vi "testingImagesROI.vi"(8 "error in (no error)":errorcluster) -> (0 "error out":errorcluster)   [LabVIEW 2017]
doc: "Use this template to build a VI to use as a subVI."
uses:
  AEROTECstageAPI/SingleStageData.ctl
  AEROTECstageAPI/StageEnum.ctl
  AEROTECstageAPI/MoveDistanceInAxis.ctl
  Utility/Axis Direction Definition.ctl
  <vilib>/event_ctls.llb/lveventtype.ctl
  <vilib>/vision/NI_Vision_Development_Module.lvlib
panel:
  out "Number of Points":i32
  in  "Point Spacing (microns)":dbl(slide)=0.2 min=0.2 max=1000.0 scale=0.0..10.0
  in  "Clear Points":bool
  in  "File Path":path=path "C:/Users/OmerLab/Documents/GitHub/RamanSpecUsingStageXY/imagesForTesting/Snap-15.jpg"
  in  "Calibration Axis Info":T1={"Origin Pixel"={"X"=1232.0, "Y"=1028.0}, "Angle Relative to Horizontal (deg)"=0.0, "Axis Reference"=0} {"Axis Reference" items=["Direct", "Indirect"]; "Angle Relative to Horizontal (deg)" format="%.2f"; "Origin Pixel"."Y" format="%.2f"; "Origin Pixel"."X" format="%.2f"}
  in  "Refresh Button":bool
  in  "Disable Stage":bool
  in  "Right Button":bool
  in  "Down Button":bool
  in  "Up Button":bool
  in  "Enable Stage":bool
  in  "Distance (mm)":dbl
  in  "Left Button":bool
  out "error out 2":errorcluster
  in  "stop 2":bool
  out "Stage Data":T2[](array[typedef])
  in  "Skip Forward Button":bool
  in  "Which point to translate?":i32
  in  "stop":bool
  out "Image":T3(plugin-control)
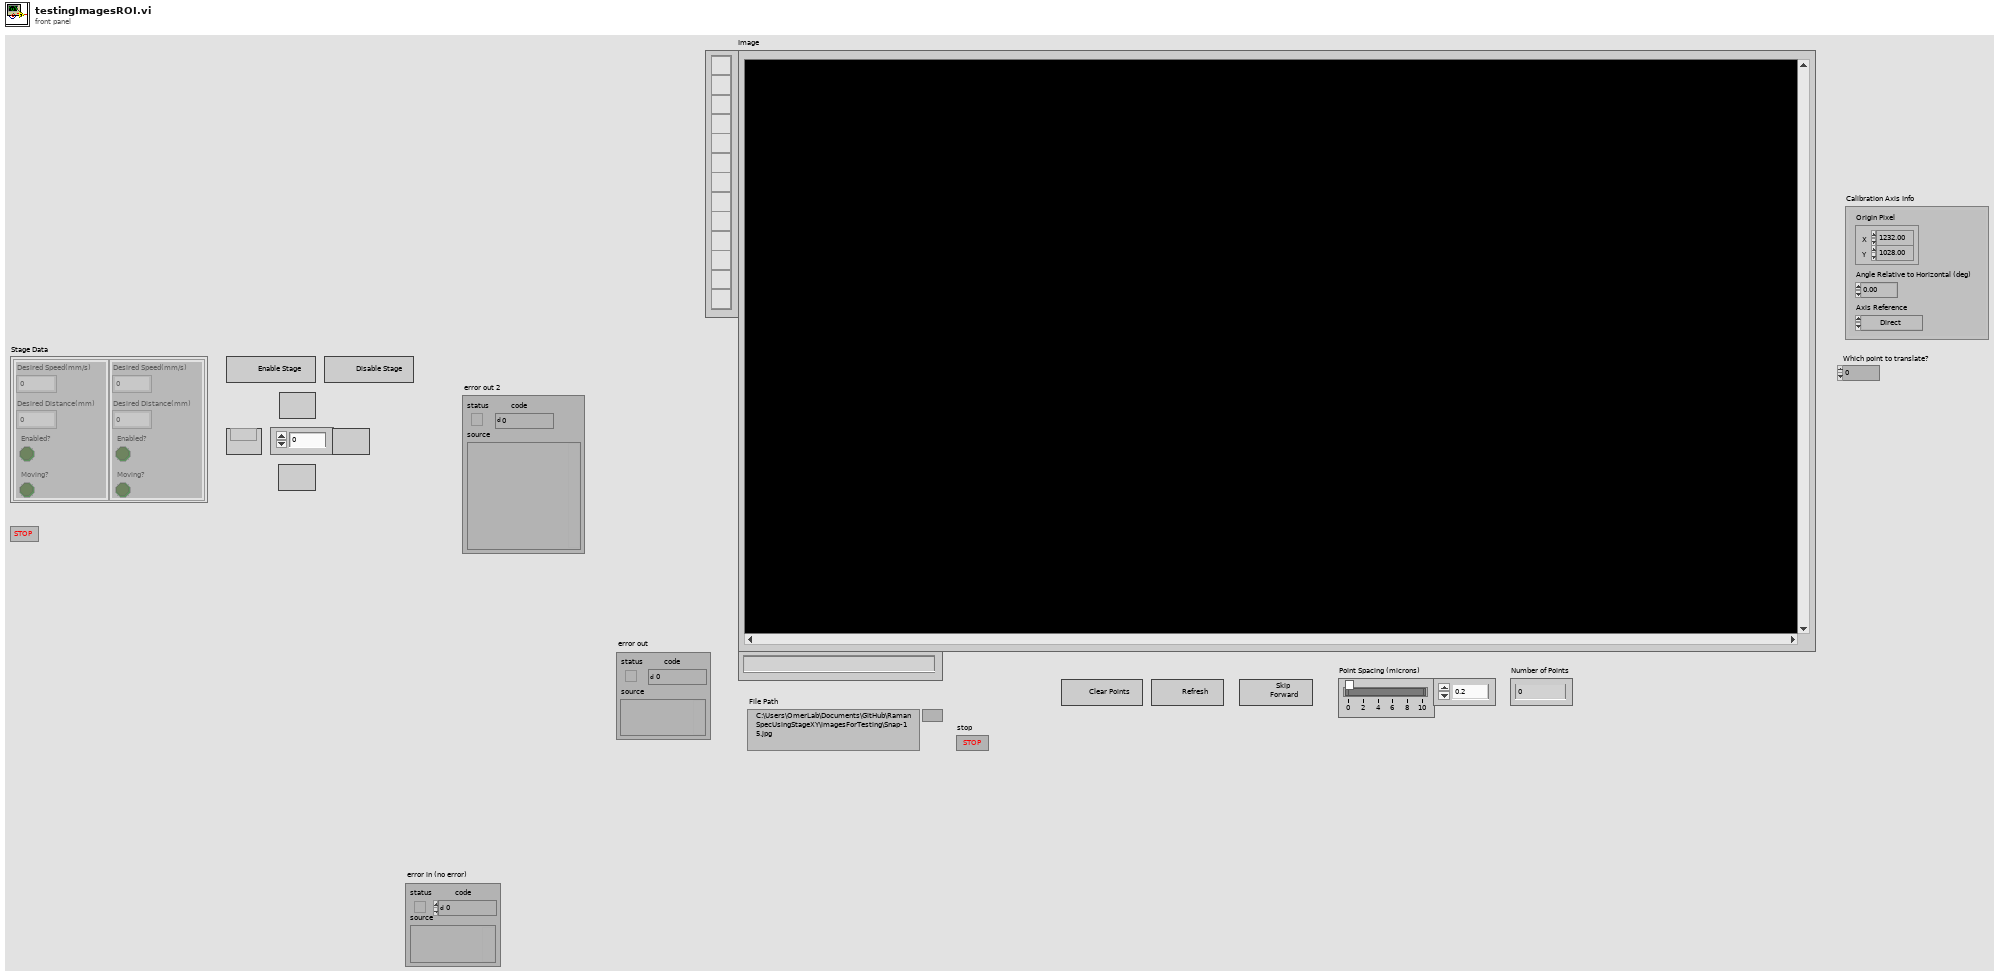
[diagram p1: front panel]
types:
  T1 = cluster{"Origin Pixel":cluster{"X":sgl, "Y":sgl}, "Angle Relative to Horizontal (deg)":sgl, "Axis Reference":u32}
  T2 = typedef "SingleStageData.ctl" = cluster{"Desired Speed(mm/s)":dbl, "Desired Distance(mm)":dbl, "Enabled?":bool, "Moving?":bool}
  T3 = typedef "IMAQ Image.ctl" = refnum<image>
  T4 = typedef "StageEnum.ctl" = enum16{"Move axis!", "Enable Stage!", "Stop Stage Controller!", "Set Default Speeds!", "Get Stage Parameters", "Start Stage Controller!", "Init"}
  T5 = typedef "lveventtype.ctl" = enum32{"Null", "Timeout", "Annotation Menu Selection", "Annotation Menu Selection?", "App Instance Close", "App Instance Close?", "Autoscale Range Change", "Bookmark Info Change", "Cell Edit", "Cell Edit?", "Cursor Grab", "Cursor Grab?", "Cursor Menu Selection", "Cursor Menu Selection?", "Cursor Move", "Cursor Release", "Data Change", "Direction Change", "Display State Change", "Drag Ended", "Drag Enter", "Drag Leave", "Drag Over", "Drag Source Update", "Drag Starting", "Drag Starting?", "Drop", "Exec State Change", "Key Down", "Key Down?", "Key Repeat", "Key Repeat?", "Key Up", "Listbox Double Click", "Menu Activation?", "Menu Selection (App)", "Menu Selection? (App)", "Menu Selection (User)", "Mouse Down", "Mouse Down?", "Mouse Enter", "Mouse Leave", "Mouse Move", "Mouse Up", "Mouse Wheel", "NI Security User Change (App)", "Pane Size", "Panel Close", "Panel Close?", "Panel Resize", "Plot Attribute Change", "Scale Range Change", "Shortcut Menu Activation?", "Shortcut Menu Selection (App)", "Shortcut Menu Selection? (App)", "Shortcut Menu Selection (User)", "Tree Double Click", "Tree Drag", "Tree Drag?", "Tree Drop", "Tree Drop?", "Tree Item Close", "Tree Item Close?", "Tree Item Open", "Tree Item Open?", "User Event", "Value Change"}
  T6 = typedef "Axis Direction Definition.ctl" = enum16{"Axis left/right", "Axis up/down"}
  T7 = typedef "MoveDistanceInAxis.ctl" = cluster{"Axis Number":i16, "Distance (microns)":dbl}
  T8 = cluster{"Global Rectangle":i32[], "Contours":cluster{"Contour Type":u32, "ROI Type":u32, "Points":i32[]}[]}
  T9 = cluster{"Contour Type":u32, "ROI Type":u32, "Points":i32[]}[]
  T10 = cluster{"Contour Type":u32, "ROI Type":u32, "Points":i32[]}
  T11 = typedef "Simple Grid Descriptor" = cluster{"X Step":sgl, "Y Step":sgl, "Unit":T12}
  T12 = typedef "Image Unit" = enum32{"Undefined", "Angström", "Micrometer", "Millimeter", "Centimeter", "Meter", "Kilometer", "Microinch", "Inch", "Feet", "Nautical miles", "Standard miles", "Steps"}
  T13 = typedef "Image Type" = u32
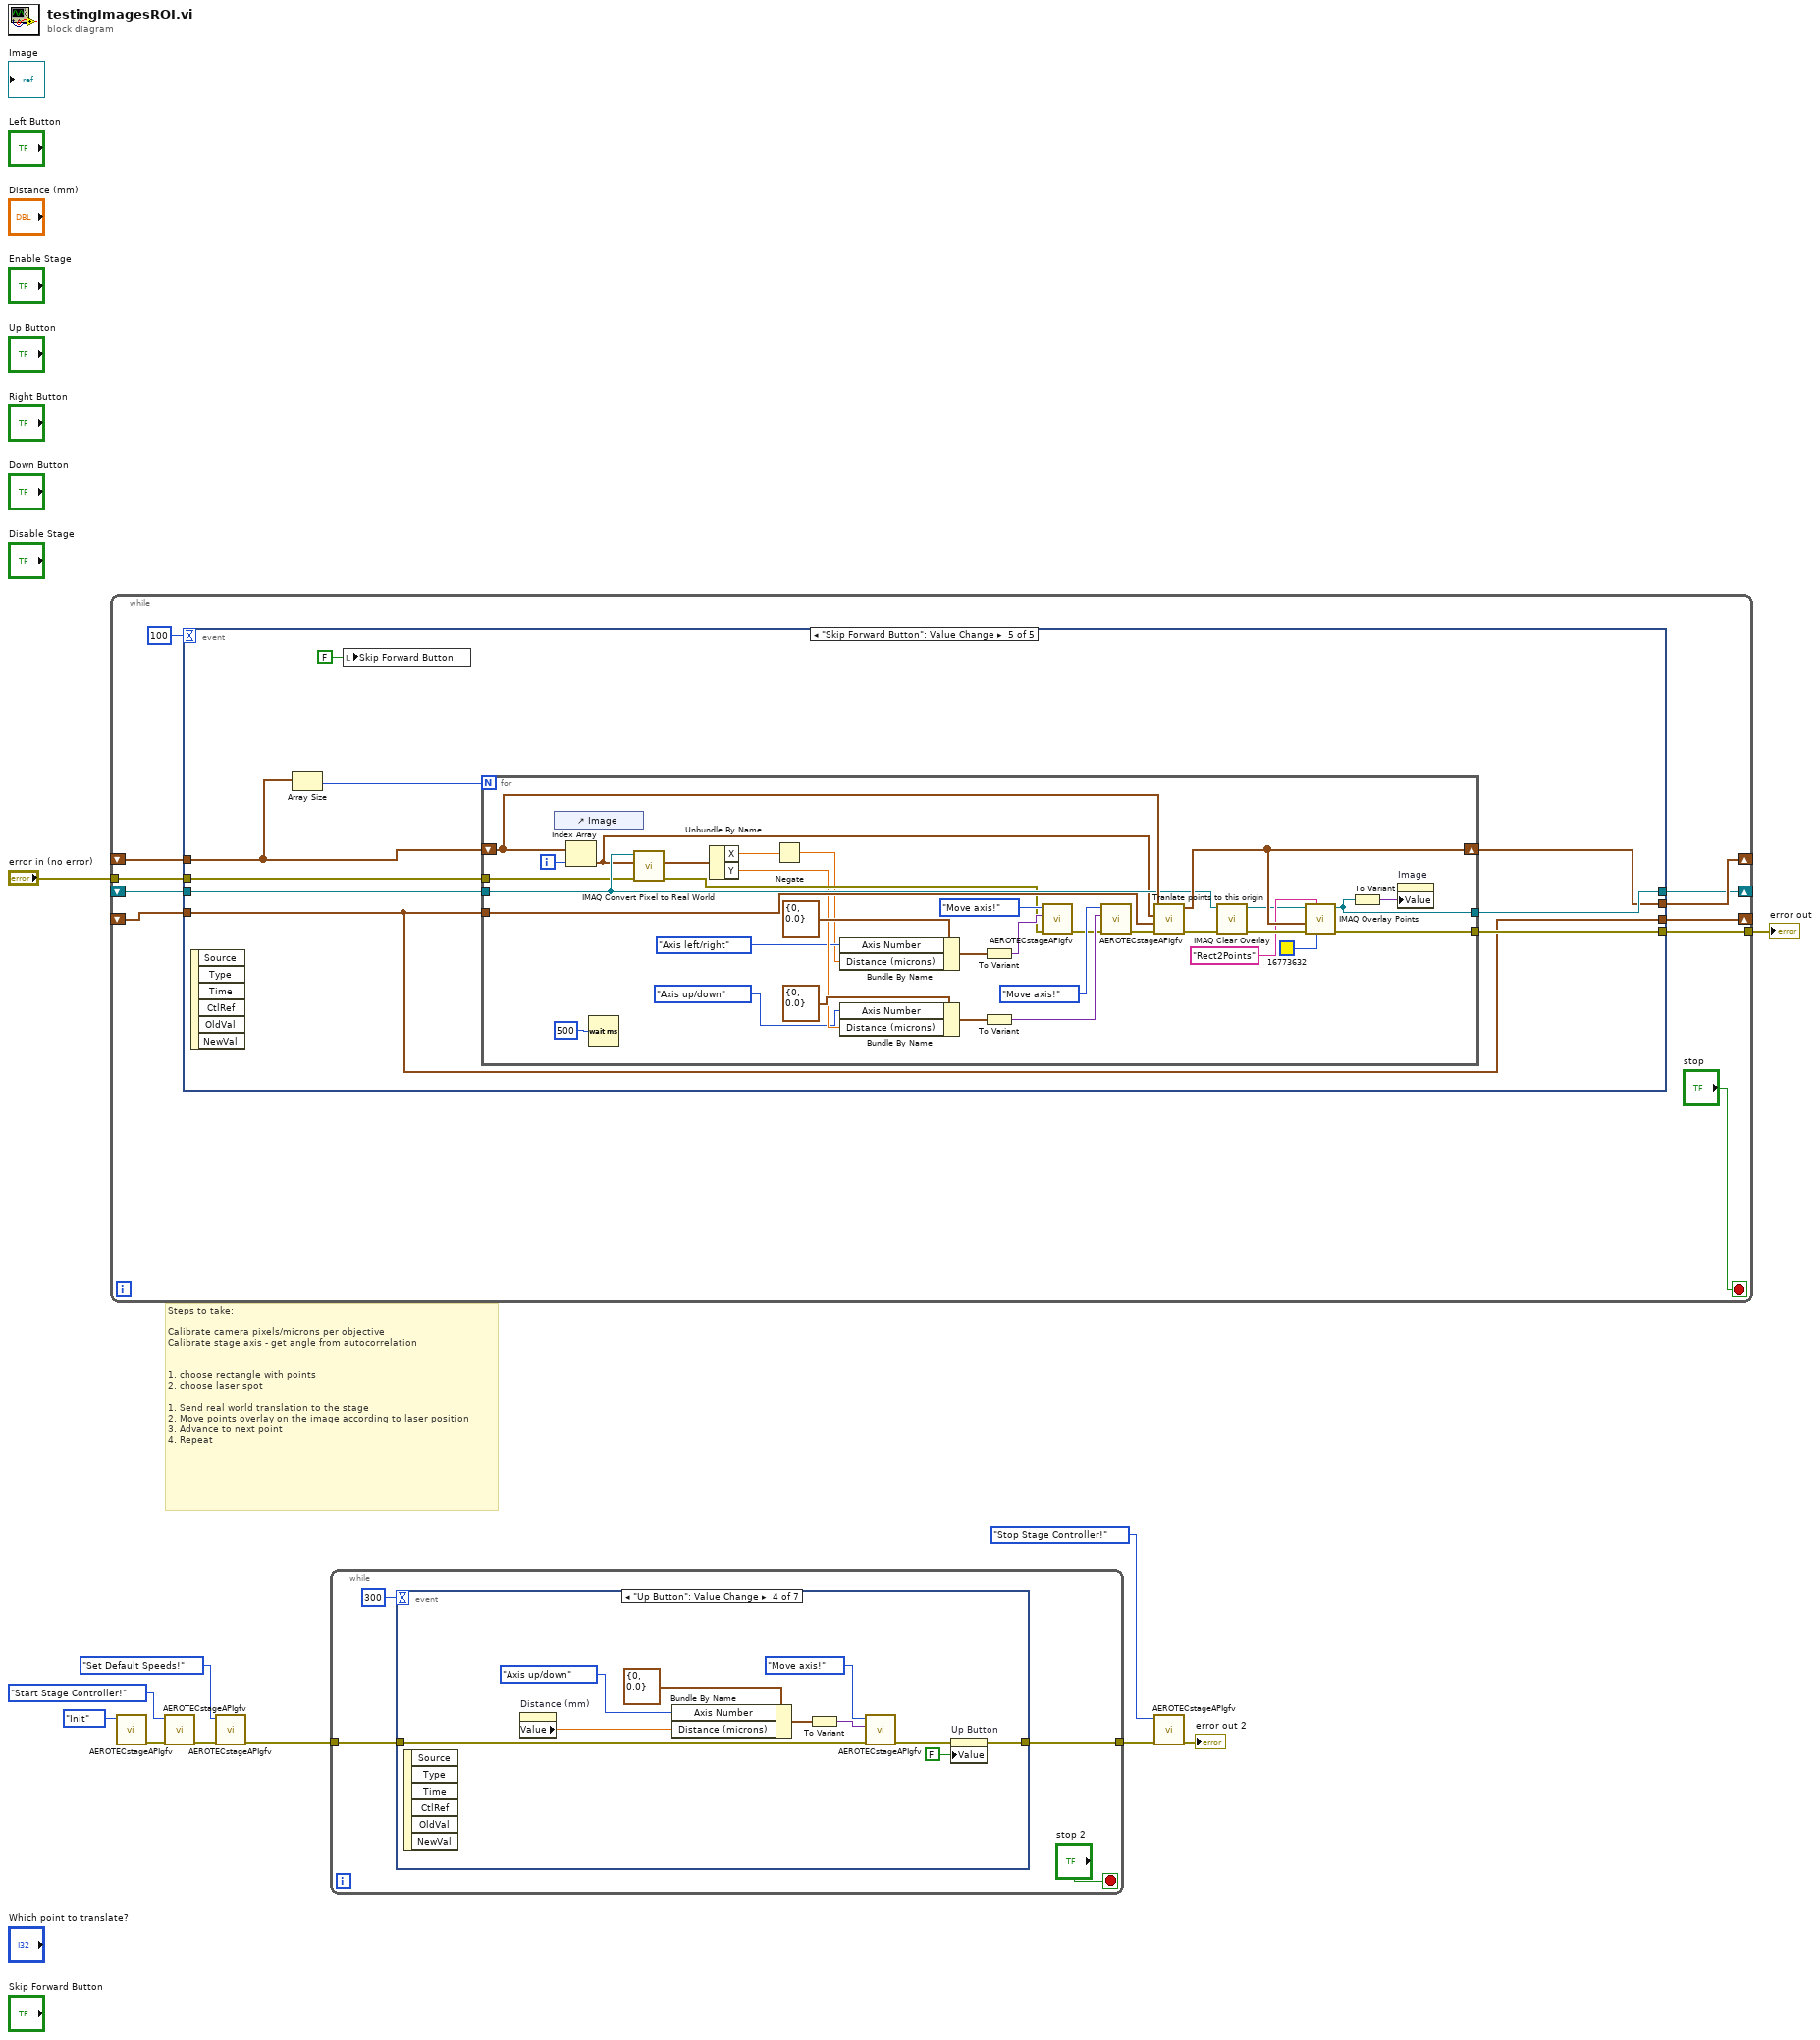
[diagram p0: block diagram]
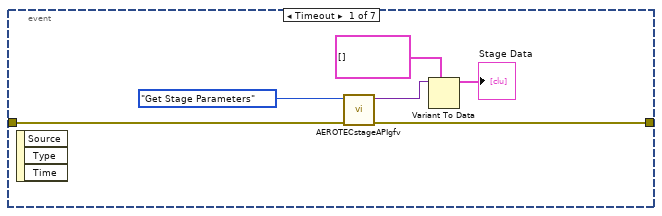
[diagram p2: hidden frame]
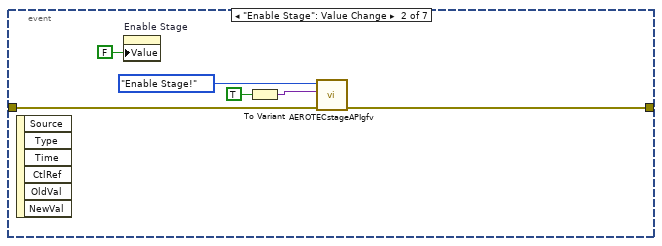
[diagram p3: hidden frame]
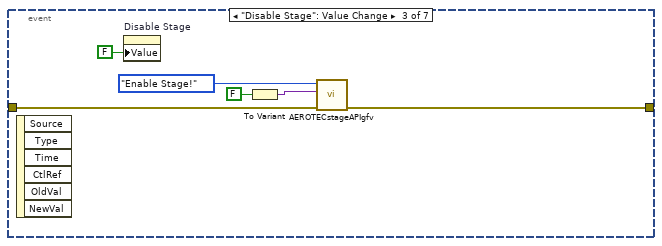
[diagram p4: hidden frame]
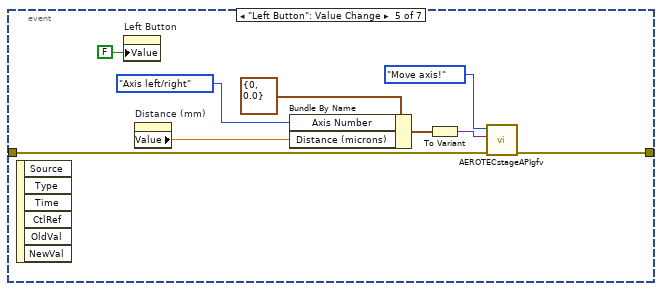
[diagram p5: hidden frame]
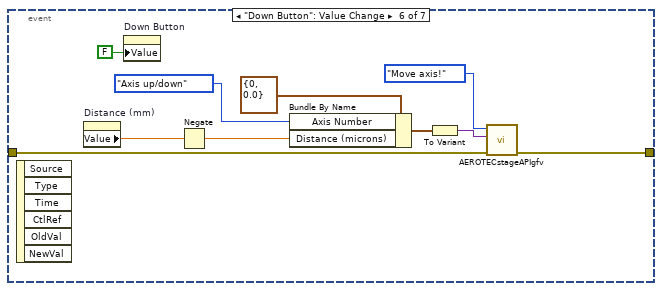
[diagram p6: hidden frame]
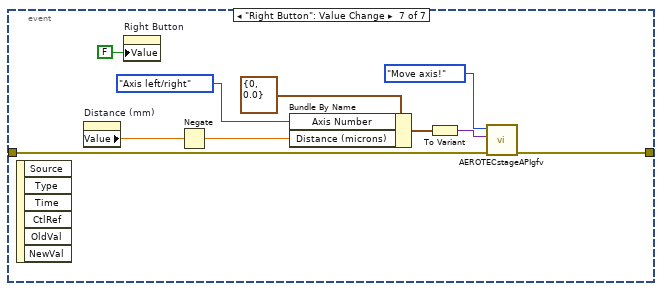
[diagram p7: hidden frame]
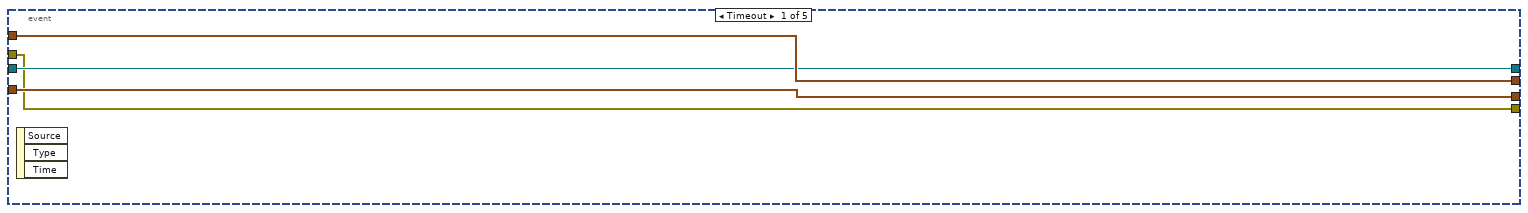
[diagram p8: hidden frame]
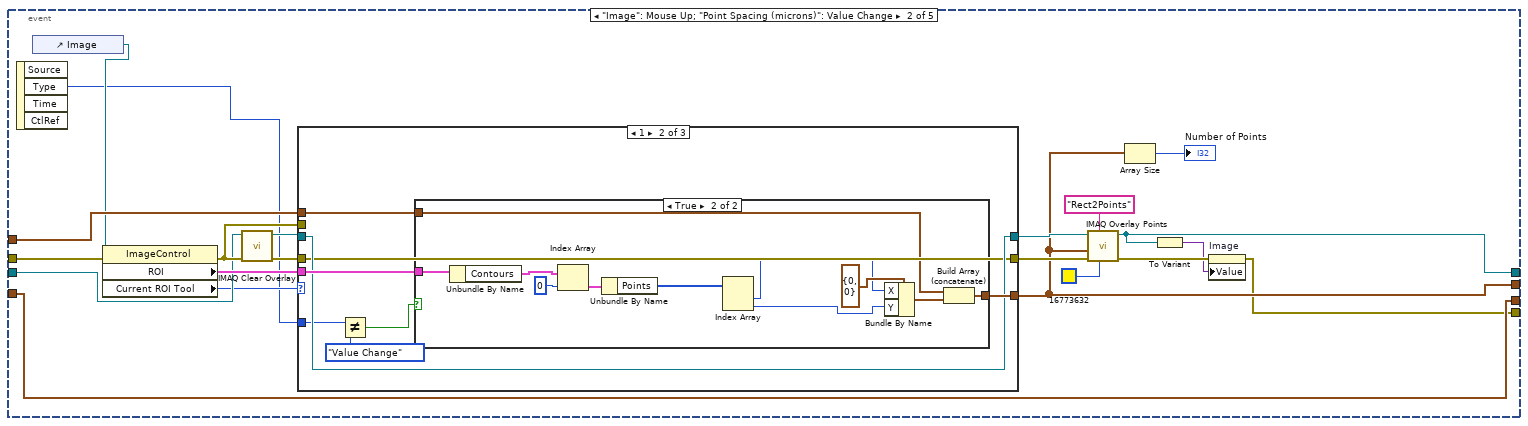
[diagram p9: hidden frame]
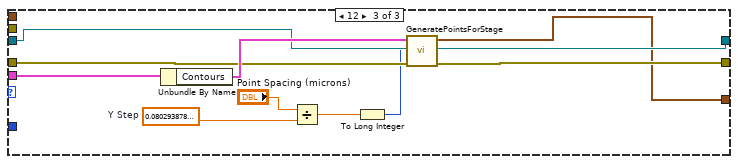
[diagram p12: hidden frame]
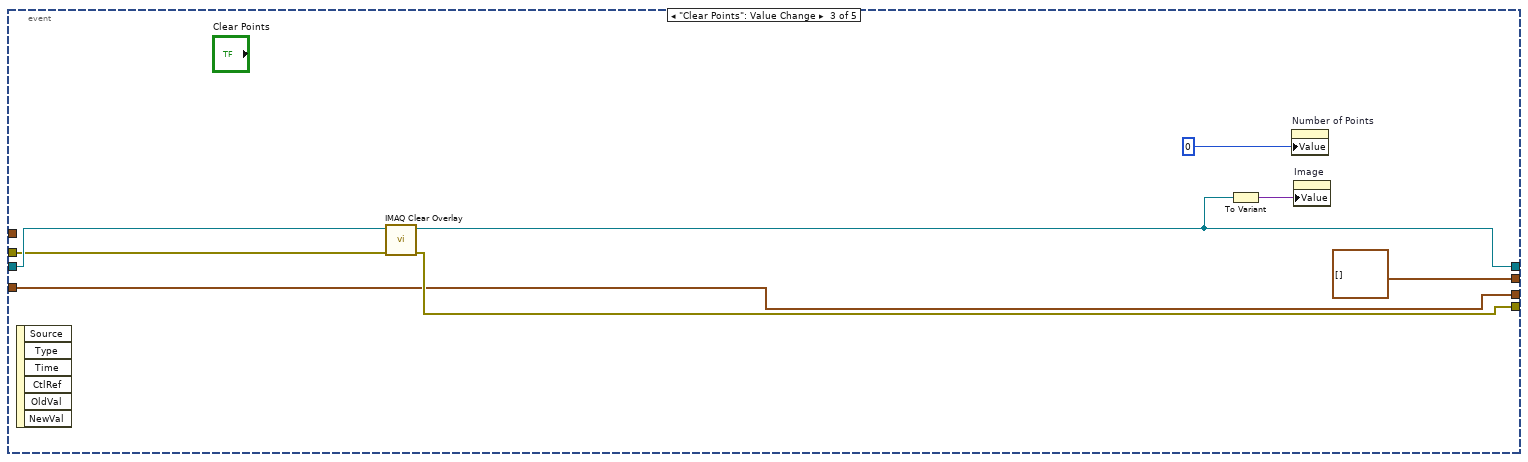
[diagram p13: hidden frame]
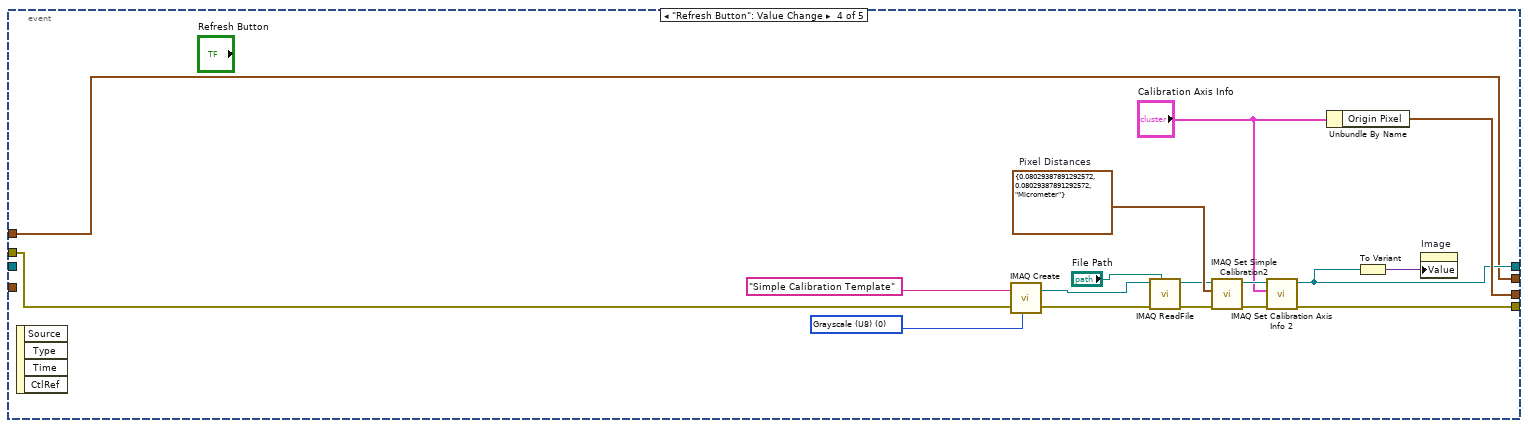
[diagram p14: hidden frame]
diagram:
  # "Steps to take:\n\nCalibrate camera pixels/microns per objective\nCalibrate stage axis - get angle from autocorrelation\n\n\n1. choose rectangle with points\n2. choose laser spot\n\n1. Send real world translation to the stage\n2. Move points overlay on the image according to laser position\n3. Advance to next point\n4. Repeat"
  n1 = while {
    tunnel: [w19] -> w11
    tunnel: "error in (no error)" -> [w18]
    shift-right: [w17] -> _
    shift-left: _ -> [w14]
    shift-right: [w16] -> _
    shift-left: _ -> [w15]
    shift-right: [w13] -> _
    shift-left: _ -> [w12]
    stop <- "stop" stop-if-true
    n2 = event shown="[4] \"Skip Forward Button\": Value Change" {
      selector: _ -> [_ _ _ _ _]
      dyn-events: _ -> [_ _ _ _ _]
      timeout: 100 -> [_ _ _ _ _]
      tunnel: [w22 w26 w84 w92 w111] -> w19
      tunnel: w18 -> [w22 w45 w85 w91 w112]
      tunnel: [w23 w44 w83 w95 w109] -> w17
      tunnel: [w25 w29 cluster{"X":i32, "Y":i32}[] [] ("Shift points") w88 w107] -> w16
      tunnel: w15 -> [w25 w40 _ w88 w106]
      tunnel: w14 -> [w23 w44 w83 _ w109]
      tunnel: [w24 w37 w81 w93 w108] -> w13
      tunnel: w12 -> [w24 w42 w86 _ w110]
      event Timeout {
        n3 = event-data() -> ()  [unwired: 1 in, 3 out]
      }
      event "Image": Mouse Up; "Point Spacing (microns)": Value Change {
        n4 = event-data() -> ("Type"=w27:T5)  [unwired: 1 in, 3 out]
        n5 = control-ref of="Image"() -> (w30:refnum<vi>)
        n6 = property class="ImageControl"(reference=w30, error in=w45) -> (error out=w43:errorcluster, "ROI"=w46:T8, "Current ROI Tool"=w41:u32)  [unwired: 1 out]
        n7 = call "IMAQ Clear Overlay"("error in (no error)"=w43, "Image"=w42) -> ("error out"=w39:errorcluster, "Image Out"=w38:T3)  [unwired: 8 in]
        n8 = case shown="1" w41 {
          tunnel: w46 -> [_ w57 w79]
          tunnel: [w47 w55 w70] -> w29
          tunnel: [w49 w54 w75] -> w31
          tunnel: w43 -> [_ _ _]
          tunnel: w40 -> [w47 w56 _]
          tunnel: w39 -> [w48 w53 w77]
          tunnel: w38 -> [w49 w54 w75]
          tunnel: [w48 w53 w76] -> w33
          tunnel: w27 -> [_ w52 _]
          frame 0, Default {
          }
          frame 1 {
            n9 = Not Equal?(x=w52, y=lveventtype."Value Change" ("Type")) -> (x != y?=w50:bool)
            n10 = case shown="True" w50 {
              tunnel: w57 -> [_ w69]
              tunnel: w56 -> [w58 w65]
              tunnel: [w58 w59] -> w55
              frame False {
              }
              frame True {
                n11 = Unbundle By Name(w69) -> ("Contours"=w68:T9)
                n12 = Index Array(array=w68, index=0) -> (element=w66:T10)
                n13 = Unbundle By Name(w66) -> ("Points"=w63:i32[])
                n14 = Index Array(array=w63) -> (element #1=w62:i32, element #2=w61:i32)  [unwired: 2 in]
                n15 = Bundle By Name(cluster=cluster{"X":i32, "Y":i32} {"X"=0, "Y"=0} ("Point Coordinates"), "X"=w62, "Y"=w61) -> (w60:cluster{"X":i32, "Y":i32})
                n16 = Build Array (concatenate)(w65, w60) -> (w59:cluster{"X":i32, "Y":i32}[])
              }
            }
          }
          frame 12 {
            w73 = sgl 0.08029388  # Y Step
            n17 = Unbundle By Name(w79) -> ("Contours"=w78:T9)
            n18 = Divide(x="Point Spacing (microns)", y=w73) -> (x/y=w72:dbl)
            n19 = To Long Integer(number=w72) -> (32bit integer=w71:i32)
            n20 = call "GeneratePointsForStage.vi"("error in (no error)"=w77, "Point Spacing"=w71, "Rotated Rect"=w78) -> ("error out"=w76:errorcluster, "PointsInRotatedRect"=w70:cluster{"X":i32, "Y":i32}[])  [unwired: 7 in]
          }
        }
        n21 = call "IMAQ Overlay Points"("Color"=u32 16773632, "Group"="Rect2Points", "error in (no error)"=w33, "Array of Points"=w29, "Image"=w31) -> ("error out"=w36:errorcluster, "Image Out"=w37:T3)  [unwired: 5 in]
        n22 = Array Size(array=w29) -> (size(s)=→"Number of Points":i32)
        n23 = To Variant(anything=w37) -> (Variant=w35:variant)
        n24 = property on="Image" class="ImageControl"(error in=w36, "Value"=w35) -> (error out=w26:errorcluster)  [unwired: 1 in, 1 out]
      }
      event "Clear Points": Value Change {
        n25 = event-data() -> ()  [unwired: 1 in, 6 out]
        n26 = call "IMAQ Clear Overlay"("error in (no error)"=w85, "Image"=w86) -> ("error out"=w84:errorcluster, "Image Out"=w81:T3)  [unwired: 8 in]
        n27 = To Variant(anything=w81) -> (Variant=w82:variant)
        n28 = property on="Number of Points" class="DigNum (strict)"("Value"=0 ("Number of Points")) -> ()  [unwired: 2 in, 2 out]
        n29 = property on="Image" class="ImageControl"("Value"=w82) -> ()  [unwired: 2 in, 2 out]
      }
      event "Refresh Button": Value Change {
        w99 = T11 {"X Step"=0.08029388, "Y Step"=0.08029388, "Unit"=enum."Micrometer"}  # Pixel Distances
        w100 = T13 0 items=["Grayscale (U8)", "Grayscale (I16)", "Grayscale (SGL)", "Complex (CSG)", "RGB (U32)", "HSL (U32)", "RGB (U64)", "Grayscale (U16)"] ("Image Type")
        n30 = event-data() -> ()  [unwired: 1 in, 4 out]
        n31 = call "IMAQ Create"("Image Name"="Simple Calibration Template", "Image Type"=w100, "error in (no error)"=w91) -> ("New Image"=w102:T3, "error out"=w104:errorcluster)  [unwired: 1 in, 1 out]
        n32 = call "IMAQ ReadFile"("File Path"="File Path", "error in (no error)"=w104, "Image"=w102) -> ("error out"=w89:errorcluster, "Image Out"=w90:T3)  [unwired: 4 in, 3 out]
        n33 = call "IMAQ Set Simple Calibration2"("error in (no error)"=w89, "Pixel Distances"=w99, "Image"=w90) -> ("error out"=w97:errorcluster, "Calibration Template Image"=w98:T3)  [unwired: 7 out]
        n34 = call-poly "IMAQ Set Calibration Axis Info 2"("error in (no error)"=w97, "Calibration Axis Info"="Calibration Axis Info", "Calibration Template Image In"=w98) -> ("error out"=w92:errorcluster, "Calibration Template Image Out"=w93:T3)  [unwired: 7 in]
        n35 = Unbundle By Name("Calibration Axis Info") -> ("Origin Pixel"=w95:cluster{"X":sgl, "Y":sgl})
        n36 = To Variant(anything=w93) -> (Variant=w94:variant)
        n37 = property on="Image" class="ImageControl"("Value"=w94) -> ()  [unwired: 2 in, 2 out]
      }
      event "Skip Forward Button": Value Change {
        n38 = event-data() -> ()  [unwired: 1 in, 6 out]
        n39 = Array Size(array=w106) -> (size(s)=w105:i32)
        n40 = local write "Skip Forward Button"(FALSE ("Skip Forward Button")) -> ()
        n41 = for {
          N: w105 -> [_]
          tunnel: w109 -> [w146]
          tunnel: w112 -> [w125]
          tunnel: [w144] -> w111
          tunnel: w110 -> [w127]
          tunnel: [w116] -> w108
          shift-right: [w143] -> w107
          shift-left: w106 -> [w137]
          i -> [w136]
          n42 = control-ref of="Image"() -> ()  [unwired: 1 out]
          n43 = Index Array(array=w137, index=w136) -> (element=w126:cluster{"X":i32, "Y":i32})
          n44 = Wait (ms)(milliseconds to wait=u32 500) -> ()  [unwired: 1 out]
          n45 = call "IMAQ Convert Pixel to Real World"("error in (no error)"=w125, "Pixel Coordinates"=w126, "Calibrated Image"=w127) -> ("error out"=w124:errorcluster, "Real World Coordinates"=w121:cluster{"X":sgl, "Y":sgl})  [unwired: 3 in, 4 out]
          n46 = Unbundle By Name(w121) -> ("X"=w115:sgl, "Y"=w120:sgl)
          n47 = Negate(x=w115) -> (-x=w114:sgl)
          n48 = Bundle By Name(cluster=T7 {"Axis Number"=0, "Distance (microns)"=0.0} ("MoveDistanceInAxis"), "Axis Number"=Axis_Direction_Definition."Axis left/right", "Distance (microns)"=w114) -> (w135:T7)
          n49 = Bundle By Name(cluster=T7 {"Axis Number"=0, "Distance (microns)"=0.0} ("MoveDistanceInAxis"), "Axis Number"=Axis_Direction_Definition."Axis up/down", "Distance (microns)"=w120) -> (w128:T7)
          n50 = To Variant(anything=w135) -> (Variant=w133:variant)
          n51 = To Variant(anything=w128) -> (Variant=w130:variant)
          n52 = call "AEROTECstageAPIgfv.vi"("error in (no error)"=w124, "Data in"=w133, 11:StageEnum."Move axis!") -> ("error out"=w123:errorcluster)  [unwired: 7 in, 1 out]
          n53 = call "AEROTECstageAPIgfv.vi"("error in (no error)"=w123, "Data in"=w130, 11:StageEnum."Move axis!") -> ("error out"=w122:errorcluster)  [unwired: 7 in, 1 out]
          n54 = call "Tranlate points to this origin.vi"("error in (no error)"=w122, "Laser Position"=w146, "New Origin Point"=w126, "Points"=w137) -> ("error out"=w141:errorcluster, "Shift points"=w143:cluster{"X":i32, "Y":i32}[])  [unwired: 4 in]
          n55 = call "IMAQ Clear Overlay"("error in (no error)"=w141, "Image"=w127) -> ("error out"=w142:errorcluster, "Image Out"=w139:T3)  [unwired: 8 in]
          n56 = call "IMAQ Overlay Points"("Color"=u32 16773632, "Group"="Rect2Points", "error in (no error)"=w142, "Array of Points"=w143, "Image"=w139) -> ("error out"=w144:errorcluster, "Image Out"=w116:T3)  [unwired: 5 in]
          n57 = To Variant(anything=w116) -> (Variant=w117:variant)
          n58 = property on="Image" class="ImageControl"("Value"=w117) -> ()  [unwired: 2 in, 2 out]
        }
      }
    }
  }
  "error out" <- w11
  n59 = call "AEROTECstageAPIgfv.vi"(11:StageEnum."Init") -> ("error out"=w8:errorcluster)  [unwired: 9 in, 1 out]
  n60 = call "AEROTECstageAPIgfv.vi"("error in (no error)"=w8, 11:StageEnum."Start Stage Controller!") -> ("error out"=w4:errorcluster)  [unwired: 8 in, 1 out]
  n61 = call "AEROTECstageAPIgfv.vi"("error in (no error)"=w4, 11:StageEnum."Set Default Speeds!") -> ("error out"=w2:errorcluster)  [unwired: 8 in, 1 out]
  n62 = while {
    tunnel: w2 -> [w148]
    tunnel: [w147] -> w1
    stop <- "stop 2" stop-if-true
    n63 = event shown="[3] \"Up Button\": Value Change" {
      selector: _ -> [_ _ _ _ _ _ _]
      dyn-events: _ -> [_ _ _ _ _ _ _]
      timeout: 300 -> [_ _ _ _ _ _ _]
      tunnel: w148 -> [w153 w162 w168 w178 w187 w197 w207]
      tunnel: [w151 w161 w167 w171 w186 w196 w206] -> w147
      event Timeout {
        n64 = event-data() -> ()  [unwired: 1 in, 3 out]
        n65 = call "AEROTECstageAPIgfv.vi"("error in (no error)"=w153, 11:StageEnum."Get Stage Parameters") -> ("error out"=w151:errorcluster, "Data Out"=w156:variant)  [unwired: 8 in]
        n66 = Variant To Data(type=T2[] [], Variant=w156) -> (data=→"Stage Data":T2[])  [unwired: 1 in, 1 out]
      }
      event "Enable Stage": Value Change {
        n67 = event-data() -> ()  [unwired: 1 in, 6 out]
        n68 = property on="Enable Stage" class="Bool (strict)"("Value"=FALSE) -> ()  [unwired: 2 in, 2 out]
        n69 = To Variant(anything=TRUE) -> (Variant=w158:variant)
        n70 = call "AEROTECstageAPIgfv.vi"("error in (no error)"=w162, "Data in"=w158, 11:StageEnum."Enable Stage!") -> ("error out"=w161:errorcluster)  [unwired: 7 in, 1 out]
      }
      event "Disable Stage": Value Change {
        n71 = event-data() -> ()  [unwired: 1 in, 6 out]
        n72 = property on="Disable Stage" class="Bool (strict)"("Value"=FALSE ("Disable Stage")) -> ()  [unwired: 2 in, 2 out]
        n73 = To Variant(anything=FALSE) -> (Variant=w164:variant)
        n74 = call "AEROTECstageAPIgfv.vi"("error in (no error)"=w168, "Data in"=w164, 11:StageEnum."Enable Stage!") -> ("error out"=w167:errorcluster)  [unwired: 7 in, 1 out]
      }
      event "Up Button": Value Change {
        n75 = event-data() -> ()  [unwired: 1 in, 6 out]
        n76 = property on="Distance (mm)" class="DigNum (strict)"() -> ("Value"=w169:dbl)  [unwired: 2 in, 2 out]
        n77 = Bundle By Name(cluster=T7 {"Axis Number"=0, "Distance (microns)"=0.0} ("MoveDistanceInAxis"), "Axis Number"=Axis_Direction_Definition."Axis up/down", "Distance (microns)"=w169) -> (w174:T7)
        n78 = To Variant(anything=w174) -> (Variant=w176:variant)
        n79 = call "AEROTECstageAPIgfv.vi"("error in (no error)"=w178, "Data in"=w176, 11:StageEnum."Move axis!") -> ("error out"=w172:errorcluster)  [unwired: 7 in, 1 out]
        n80 = property on="Up Button" class="Bool (strict)"(error in=w172, "Value"=FALSE ("Disable Stage")) -> (error out=w171:errorcluster)  [unwired: 1 in, 1 out]
      }
      event "Left Button": Value Change {
        n81 = event-data() -> ()  [unwired: 1 in, 6 out]
        n82 = property on="Left Button" class="Bool (strict)"("Value"=FALSE ("Disable Stage")) -> ()  [unwired: 2 in, 2 out]
        n83 = property on="Distance (mm)" class="DigNum (strict)"() -> ("Value"=w179:dbl)  [unwired: 2 in, 2 out]
        n84 = Bundle By Name(cluster=T7 {"Axis Number"=0, "Distance (microns)"=0.0} ("MoveDistanceInAxis"), "Axis Number"=Axis_Direction_Definition."Axis left/right", "Distance (microns)"=w179) -> (w182:T7)
        n85 = To Variant(anything=w182) -> (Variant=w184:variant)
        n86 = call "AEROTECstageAPIgfv.vi"("error in (no error)"=w187, "Data in"=w184, 11:StageEnum."Move axis!") -> ("error out"=w186:errorcluster)  [unwired: 7 in, 1 out]
      }
      event "Down Button": Value Change {
        n87 = event-data() -> ()  [unwired: 1 in, 6 out]
        n88 = property on="Distance (mm)" class="DigNum (strict)"() -> ("Value"=w189:dbl)  [unwired: 2 in, 2 out]
        n89 = property on="Down Button" class="Bool (strict)"("Value"=FALSE ("Disable Stage")) -> ()  [unwired: 2 in, 2 out]
        n90 = Negate(x=w189) -> (-x=w188:dbl)
        n91 = Bundle By Name(cluster=T7 {"Axis Number"=0, "Distance (microns)"=0.0} ("MoveDistanceInAxis"), "Axis Number"=Axis_Direction_Definition."Axis up/down", "Distance (microns)"=w188) -> (w192:T7)
        n92 = To Variant(anything=w192) -> (Variant=w194:variant)
        n93 = call "AEROTECstageAPIgfv.vi"("error in (no error)"=w197, "Data in"=w194, 11:StageEnum."Move axis!") -> ("error out"=w196:errorcluster)  [unwired: 7 in, 1 out]
      }
      event "Right Button": Value Change {
        n94 = event-data() -> ()  [unwired: 1 in, 6 out]
        n95 = property on="Distance (mm)" class="DigNum (strict)"() -> ("Value"=w199:dbl)  [unwired: 2 in, 2 out]
        n96 = property on="Right Button" class="Bool (strict)"("Value"=FALSE ("Disable Stage")) -> ()  [unwired: 2 in, 2 out]
        n97 = Negate(x=w199) -> (-x=w198:dbl)
        n98 = Bundle By Name(cluster=T7 {"Axis Number"=0, "Distance (microns)"=0.0} ("MoveDistanceInAxis"), "Axis Number"=Axis_Direction_Definition."Axis left/right", "Distance (microns)"=w198) -> (w202:T7)
        n99 = To Variant(anything=w202) -> (Variant=w204:variant)
        n100 = call "AEROTECstageAPIgfv.vi"("error in (no error)"=w207, "Data in"=w204, 11:StageEnum."Move axis!") -> ("error out"=w206:errorcluster)  [unwired: 7 in, 1 out]
      }
    }
  }
  n101 = call "AEROTECstageAPIgfv.vi"("error in (no error)"=w1, 11:StageEnum."Stop Stage Controller!") -> ("error out"=→"error out 2":errorcluster)  [unwired: 8 in, 1 out]
